vi "CamCloseDeinit.vi"(8 "error in (no error)":errorcluster, 11 "hCam":i16) -> (0 "error out":errorcluster)   [LabVIEW 2021]
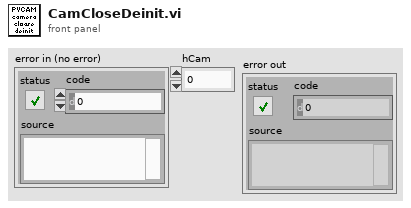
[diagram p1: front panel]
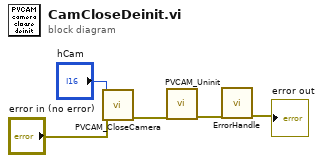
[diagram p0: block diagram]
diagram:
  n1 = call "PVCAM_CloseCamera.vi"("error in (no error)"="error in (no error)", "hCam"="hCam") -> ("error out"=w4:errorcluster)  [unwired: 8 in, 1 out]
  n2 = call "PVCAM_Uninit.vi"("error in (no error)"=w4) -> ("error out"=w2:errorcluster)  [unwired: 9 in, 1 out]
  n3 = call "ErrorHandle.vi"("error in (no error)"=w2) -> ("error in (no error) 2"=→"error out":errorcluster)  [unwired: 10 in]
